vi "TemperaturSimulation.vi"() -> ()   [LabVIEW 2020]
panel:
  out "Signalverlaufsdiagramm":dynamicdata(graph)
  in  "Format-String":string
  in  "Pfad":path=path "C:/Users/Messlabor_Kustos/Desktop/test.xls"
  in  "?":dbl
  in  "Stopp":bool
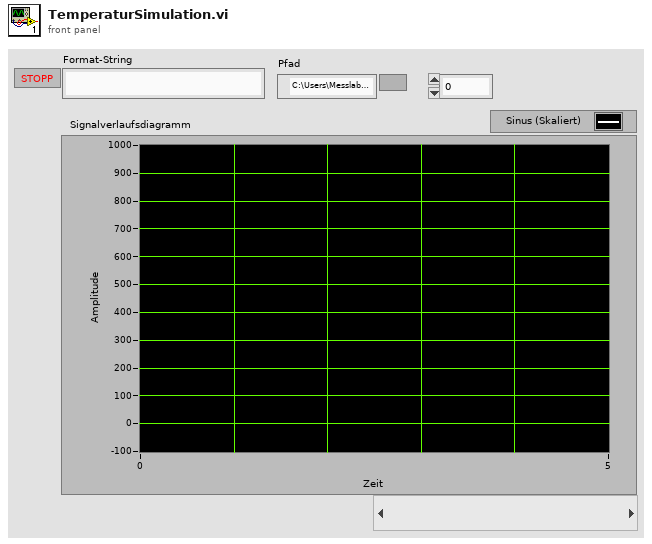
[diagram p1: front panel]
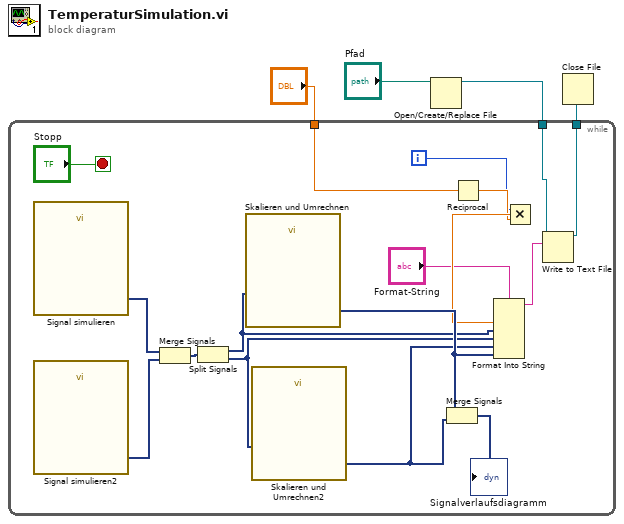
[diagram p0: block diagram]
diagram:
  n1 = Open/Create/Replace File(file path (use dialog)="Pfad") -> (refnum out=w3:refnum<file>)  [unwired: 5 in, 2 out]
  n2 = while {
    tunnel: [w11] -> w4
    tunnel: w3 -> [w10]
    tunnel: "?" -> [w5]
    i -> [w6]
    stop <- "Stopp" stop-if-true
    n3 = call "Signal simulieren"() -> ("Sinus"=w20:dynamicdata)  [unwired: 14 in, 1 out]
    n4 = call "Signal simulieren2"() -> ("Sinus"=w19:dynamicdata)  [unwired: 14 in, 1 out]
    n5 = Merge Signals(w20, w19) -> (w18:dynamicdata)
    n6 = Split Signals(w18) -> (w15:dynamicdata, w14:dynamicdata)  [unwired: 2 in]
    n7 = call "Skalieren und Umrechnen"("Signals"=w15) -> ("Scaled Signals"=w17:dynamicdata)  [unwired: 9 in, 1 out]
    n8 = call "Skalieren und Umrechnen2"("Signals"=w14) -> ("Scaled Signals"=w16:dynamicdata)  [unwired: 9 in, 1 out]
    n9 = Merge Signals(w17, w16) -> (→"Signalverlaufsdiagramm":dynamicdata)
    n10 = Reciprocal(x=w5) -> (1/x=w7:dbl)
    n11 = Multiply(x=w6, y=w7) -> (x*y=w13:dbl)
    n12 = Format Into String(format string="Format-String", w13, w15, w14, w16, w17) -> (resulting string=w12:string)  [unwired: 2 in, 1 out]
    n13 = Write to Text File(file (use dialog)=w10, text=w12) -> (refnum out=w11:refnum<file>)  [unwired: 2 in, 2 out]
  }
  n14 = Close File(refnum=w4) -> ()  [unwired: 1 in, 2 out]
